vi "Drive Controller.vi"(8 "error in":errorcluster) -> ()   [LabVIEW 2017]
doc: "This VI executes continuously carrying out the current operation and responding to updates or new operation requests. It will often contain the timing or control code that is difficult to place directly in TeleOp. This VI generally opens all sensors and motors and isolates the rest of the robot code from knowing implementation details of how the operations are carried out."
uses:
  <vilib>/Rock Robotics/WPI/Framework/Completion Status.ctl
  Drive Setpoints.ctl
  Drive Operations.ctl
  <vilib>/Rock Robotics/WPI/SafetyOutput/WPI_SafetyOutputConfigMenu.ctl
  <vilib>/Rock Robotics/SystemInterfaces/DIO/FPGA_DIOPWMChannel.ctl
  <vilib>/Rock Robotics/SystemInterfaces/DIO/FPGA_DIOChannel.ctl
  <vilib>/Rock Robotics/WPI/RobotDrive/WPI_RobotDriveOpen2MotorWithTalon.vi
  <vilib>/Rock Robotics/WPI/Counter/WPI_CounterDigitalInputToDigitalSource.vi
  gyroNumControl.vi
  <vilib>/addons/control/pid/pid.llb/PID (DBL).vi
  <vilib>/Rock Robotics/WPI/Joystick/WPI_JoystickArcadeMapping.vi
  <vilib>/addons/control/pid/NI_PID_pid.lvlib
panel:
  in  "PID Gains (DriveDistance)":T1={"proportional gain (Kc)"=1.0, "integral time (Ti, min)"=0.01, "derivative time (Td, min)"=0.0} {"derivative time (Td, min)" format="%.3f"; "integral time (Ti, min)" format="%.3f"; "proportional gain (Kc)" format="%.3f"}
  in  "PID Gains (TurnAngle)":T1={"proportional gain (Kc)"=1.0, "integral time (Ti, min)"=0.01, "derivative time (Td, min)"=0.0} {"derivative time (Td, min)" format="%.3f"; "integral time (Ti, min)" format="%.3f"; "proportional gain (Kc)" format="%.3f"}
  in  "PID gains (GuidedDrive)":T1={"proportional gain (Kc)"=0.1, "integral time (Ti, min)"=0.0, "derivative time (Td, min)"=0.0} {"derivative time (Td, min)" format="%.3f"; "integral time (Ti, min)" format="%.3f"; "proportional gain (Kc)" format="%.3f"}
  in  "Interactive Values":T2
  in  "Buttons":cluster{"Execute Cmd":bool, "Abort Cmd":bool}
  out "Command Timing":cluster{"Start Time (ms)":u32, "Iterations":i32}
  out "Status":T4
  out "Setpoints":T5(graph)
  out "Current\nCmd":string
  # "Tip: The graph shows the motor setpoints. It may also be helpful to observe inputs and sensor values.\nYou may also want to display tuning or debugging controls."
  # "Interactive Command: You may fill in the settings for a command\nand schedule it with the Execute button. You can observe and abort\nany command while fine tuning the code for the controller."
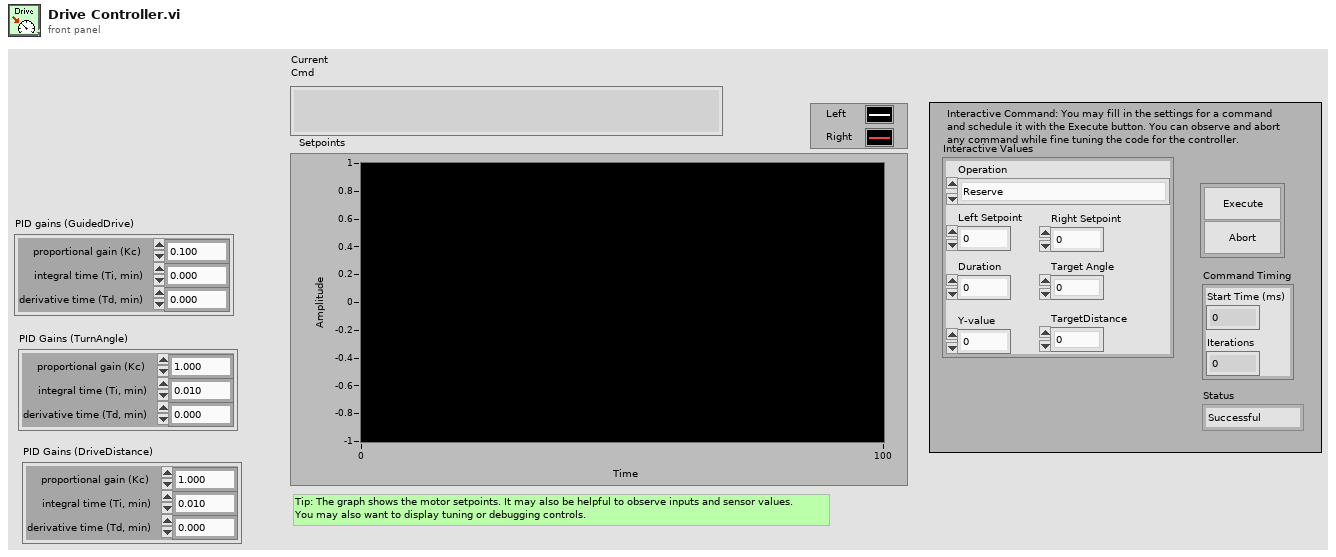
[diagram p1: front panel]
types:
  T1 = cluster{"proportional gain (Kc)":dbl, "integral time (Ti, min)":dbl, "derivative time (Td, min)":dbl}
  T2 = typedef "Drive Setpoints.ctl" = cluster{"Operation":T3, "Left Setpoint":dbl, "Right Setpoint":dbl, "Duration":dbl, "Target Angle":dbl, "Y-value":dbl, "TargetDistance":dbl}
  T3 = typedef "Drive Operations.ctl" = enum16{"Reserve", "Read Current", "Freestyle", "Drive for Distance", "TurnAngle", "Guided Drive"}
  T4 = typedef "Completion Status.ctl" = enum16{"Successful", "Aborted", "Incomplete"}
  T5 = cluster{"Left Setpoint":dbl, "Right Setpoint":dbl}
  T6 = typedef "FPGA_DIOChannel.ctl" = enum8{"DIO 0", "DIO 1", "DIO 2", "DIO 3", "DIO 4", "DIO 5", "DIO 6", "DIO 7", "DIO 8", "DIO 9", "DIO MXP 0", "DIO MXP 1", "DIO MXP 2", "DIO MXP 3", "DIO MXP 4", "DIO MXP 5", "DIO MXP 6", "DIO MXP 7", "DIO MXP 8", "DIO MXP 9", "DIO MXP 10", "DIO MXP 11", "DIO MXP 12", "DIO MXP 13", "DIO MXP 14", "DIO MXP 15", "SPI Port CS1", "SPI Port CS2", "SPI Port CS3", "SPI Port MISO", "SPI Port MOSI", "Invalid"}
  T7 = typedef "FPGA_DIOPWMChannel.ctl" = enum8{"PWM 0", "PWM 1", "PWM 2", "PWM 3", "PWM 4", "PWM 5", "PWM 6", "PWM 7", "PWM 8", "PWM 9", "PWM MXP 0", "PWM MXP 1", "PWM MXP 2", "PWM MXP 3", "PWM MXP 4", "PWM MXP 5", "PWM MXP 6", "PWM MXP 7", "PWM MXP 8", "PWM MXP 9", "Invalid"}
  T8 = typedef "WPI_SafetyOutputConfigMenu.ctl" = enum16{"Enable", "Disable"}
  T9 = typedef "WPI_DigitalInputDevRef.ctl" = cluster{"DevStatus":errorcluster, "DIO Channel":T6}
  T10 = typedef "FPGA_CounterEncoderSourceConvertionLVSourceType.ctl" = cluster{"DevStatus":errorcluster, "AnalogTriggerMode?":bool, "DigitalMode":cluster{"DIO Channel":T11}, "AnalogTriggerMode":cluster{"AnalogTriggerIndex":T12, "OutputType":T13}}
  T11 = typedef "FPGA_DIODigitalSourceChannel.ctl" = enum8{"DIO 0", "DIO 1", "DIO 2", "DIO 3", "DIO 4", "DIO 5", "DIO 6", "DIO 7", "DIO 8", "DIO 9", "DIO MXP 0", "DIO MXP 1", "DIO MXP 2", "DIO MXP 3", "DIO MXP 4", "DIO MXP 5", "DIO MXP 6", "DIO MXP 7", "DIO MXP 8", "DIO MXP 9", "DIO MXP 10", "DIO MXP 11", "DIO MXP 12", "DIO MXP 13", "DIO MXP 14", "DIO MXP 15", "Disabled"}
  T12 = typedef "FPGA_AnalogTriggerIndex.ctl" = enum8{"Trig 0", "Trig 1", "Trig 2", "Trig 3", "Trig 4", "Trig 5", "Trig 6", "Trig 7", "Invalid"}
  T13 = typedef "FPGA_AnalogTriggerOutType.ctl" = enum16{"InWindow", "TriggerState", "Rising", "Falling"}
  T14 = typedef "WPI_RobotDriveDevRef.ctl" = cluster{"DevStatus":errorcluster, "Motors[]":T15[], "Square Inputs":bool, "Max Output":dbl}
  T15 = typedef "WPI_MotorControlDeviceRef.ctl" = cluster{"DeviceStatus":errorcluster, "Type":T16, "PWM":cluster{"PWM Channel":T7, "DeadBand":T17}, "CAN":cluster{"Device Number":u8, "SetOutput VI Ref":variant, "GetOutput VI Ref":variant, "Enable VI Ref":variant, "Disable VI Ref":variant, "Data":variant}, "Invert":bool, "DIO PWM":cluster{"PWM \"Enable\" Channel":T7, "DIOChannel":T6, "PWM Rate":dbl}}
  T16 = typedef "WPI_MotorControlType.ctl" = enum16{"PWM", "CAN", "DIO PWM"}
  T17 = typedef "WPI_PWMDeadband.ctl" = cluster{"Name":string, "maxPositivePwm":i32, "minPositivePwm":i32, "centerPwm":i32, "maxNegativePwm":i32, "minNegativePwm":i32, "angularRange":u16}
  T18 = typedef "WPI_EncoderDevRef.ctl" = cluster{"DevStatus":errorcluster, "EncoderIndex":T19, "CounterIndex":T20, "DistancePerCount":dbl, "Decoding Type":T21}
  T19 = typedef "FPGA_EncoderIdx.ctl" = enum8{"Enc 0", "Enc 1", "Enc 2", "Enc 3", "Enc 4", "Enc 5", "Enc 6", "Enc 7", "Invalid"}
  T20 = typedef "FPGA_CounterCtrSystemIndex.ctl" = enum8{"Ctr 0", "Ctr 1", "Ctr 2", "Ctr 3", "Ctr 4", "Ctr 5", "Ctr 6", "Ctr 7", "Invalid"}
  T21 = typedef "WPI_EncoderType.ctl" = enum16{"1x", "2x", "4x"}
  T22 = typedef "Command Status Info.ctl" = cluster{"Name":string, "Status":T4, "notifier out":T23}
  T23 = typedef "Completion Notifier.ctl" = refnum<notifier>
  T24 = cluster{"SubSystem Data":T2, cluster{"Start Time (ms)":u32, "Iterations":i32}, cluster{"Command Info":T22, "Description":string, "Default Command":T2, "queue out":refnum<queue>, "Subsystem Name":string}}
  T25 = cluster{"SubSystem Data":T2, cluster{"Start Time (ms)":u32, "Iterations":i32}, "Default Command Arguments":cluster{"Command Info":T22, "Description":string, "Default Command":T2, "queue out":refnum<queue>, "Subsystem Name":string}}
  T26 = cluster{"Left Motor Value":dbl, "Right Motor Value":dbl}
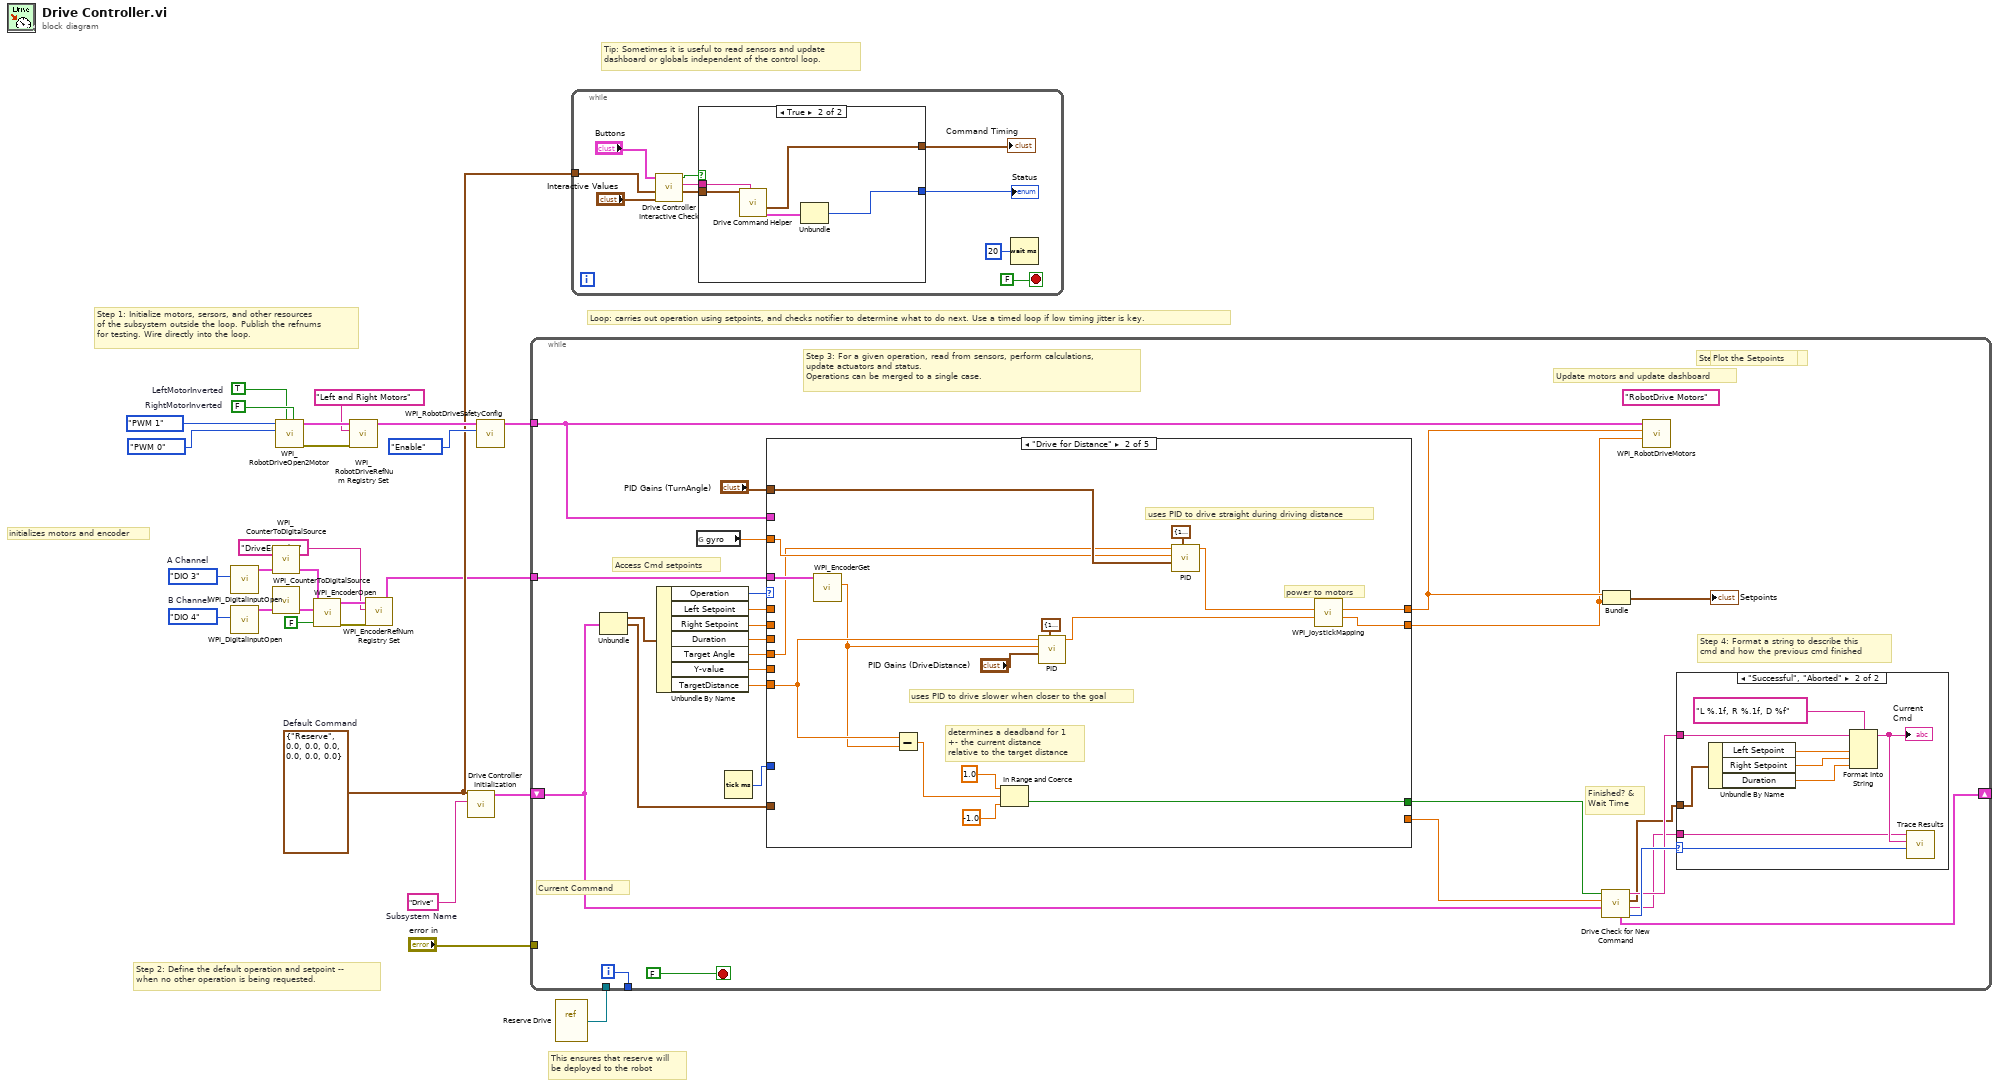
[diagram p0: block diagram]
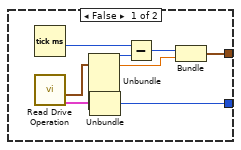
[diagram p2: hidden frame]
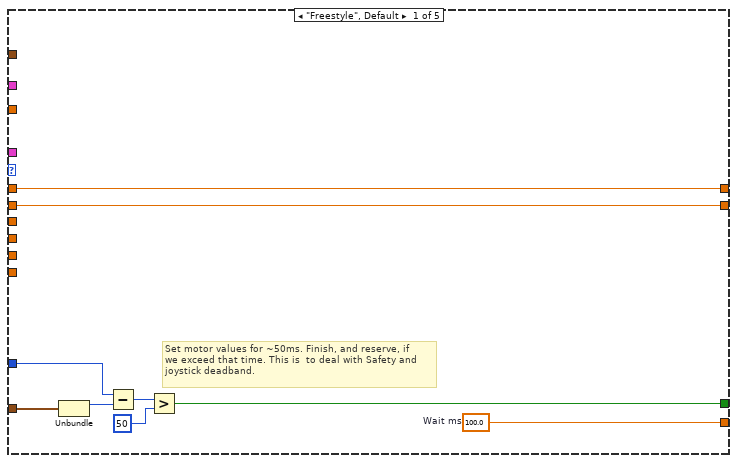
[diagram p4: hidden frame]
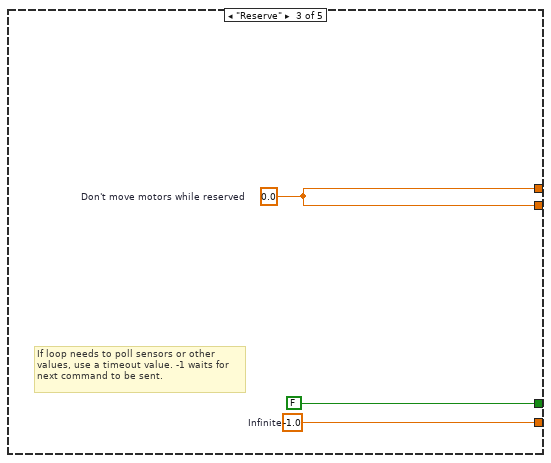
[diagram p5: hidden frame]
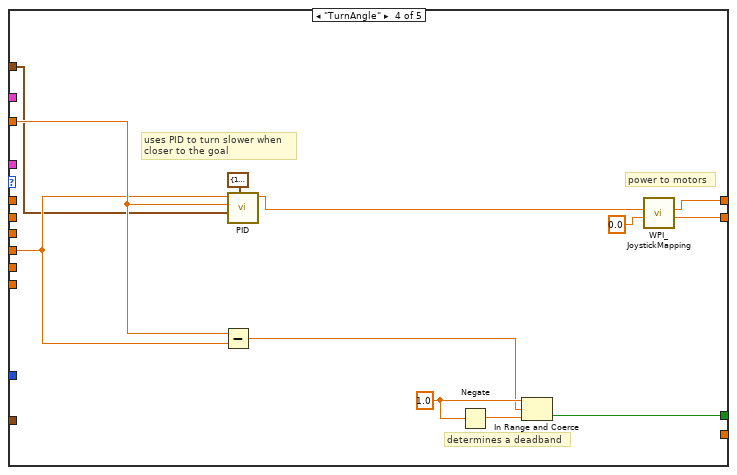
[diagram p6: hidden frame]
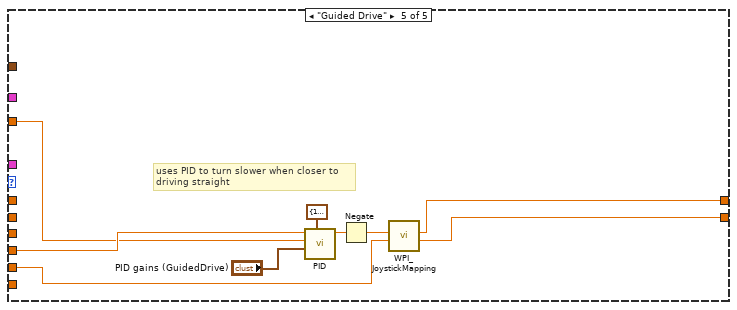
[diagram p7: hidden frame]
diagram:
  w11 = FPGA_DIOChannel."DIO 4"  # B Channel
  w10 = FPGA_DIOChannel."DIO 3"  # A Channel
  w24 = TRUE  # LeftMotorInverted
  w25 = FALSE  # RightMotorInverted
  w12 = T2 {"Operation"=enum."Reserve", "Left Setpoint"=0.0, "Right Setpoint"=0.0, "Duration"=0.0, "Target Angle"=0.0, "Y-value"=0.0, "TargetDistance"=0.0}  # Default Command
  w26 = "Drive"  # Subsystem Name
  # "initializes motors and encoder"
  # "This ensures that reserve will\nbe deployed to the robot"
  # "Tip: Sometimes it is useful to read sensors and update\ndashboard or globals independent of the control loop."
  # "Step 2: Define the default operation and setpoint --\nwhen no other operation is being requested."
  # "Step 1: Initialize motors, sersors, and other resources\nof the subsystem outside the loop. Publish the refnums\nfor testing. Wire directly into the loop."
  # "Loop: carries out operation using setpoints, and checks notifier to determine what to do next. Use a timed loop if low timing jitter is key."
  n1 = call <vilib>:"WPI_DigitalInputOpen.vi"("DIO Channel"=w10) -> ("DigitalInputDevRef"=w7:T9)  [unwired: 1 in, 9 out]
  n2 = call <vilib>:"WPI_DigitalInputOpen.vi"("DIO Channel"=w11) -> ("DigitalInputDevRef"=w8:T9)  [unwired: 1 in, 9 out]
  n3 = call-poly <vilib>:"WPI_CounterToDigitalSource.vi"("DigitalInputDevRef"=w7) -> ("Digital Source"=w6:T10)  [unwired: 6 out]
  n4 = call-poly <vilib>:"WPI_CounterToDigitalSource.vi"("DigitalInputDevRef"=w8) -> ("Digital Source"=w9:T10)  [unwired: 6 out]
  n5 = call-poly <vilib>:"WPI_RobotDriveOpen2Motor.vi"("Right Motor Inverted"=w25, "Left Motor Inverted"=w24, "Right Motor"=FPGA_DIOPWMChannel."PWM 0", "Left Motor"=FPGA_DIOPWMChannel."PWM 1") -> ("error out"=w21:errorcluster, "RobotDriveDevRef"=w23:T14)  [unwired: 1 in, 5 out]
  n6 = call <vilib>:"WPI_EncoderOpen.vi"("Invert Direction (False)"=FALSE, "BSource"=w9, "ASource"=w6) -> ("error out"=w4:errorcluster, "EncoderDevRef"=w3:T18)  [unwired: 5 in, 2 out]
  n7 = call <vilib>:"WPI_RobotDriveRefNum Registry Set.vi"("error in (no error)"=w21, "refnum name"="Left and Right Motors", "RobotDriveDevRef"=w23) -> ("RobotDriveDevRef"=w20:T14)  [unwired: 1 in, 7 out]
  n8 = call <vilib>:"WPI_EncoderRefNum Registry Set.vi"("error in (no error)"=w4, "refnum name"="DriveEncoder", "EncoderDevRef"=w3) -> ("EncoderDevRef"=w2:T18)  [unwired: 7 in, 1 out]
  n9 = call "Drive Controller Initialization.vi"("Subsystem Name"=w26, "Default Command"=w12) -> ("Current Command"=w16:T24)  [unwired: 9 in]
  n10 = call <vilib>:"WPI_RobotDriveSafetyConfig.vi"("mode"=WPI_SafetyOutputConfigMenu."Enable", "RobotDriveDevRef"=w20) -> ("RobotDriveDevRef"=w18:T14)  [unwired: 8 in, 1 out]
  n11 = vi-ref "Reserve Drive.vi"() -> (w15:refnum<vi>)
  n12 = while {
    shift-right: [w41] -> _
    shift-left: w16 -> [w35]
    tunnel: [w52] -> _
    tunnel: w18 -> [w34]
    tunnel: "error in" -> [_]
    tunnel: w15 -> [_]
    tunnel: w2 -> [w29]
    i -> [w52]
    stop <- FALSE stop-if-true
    (unwired) "RobotDrive Motors" ("Name")
    # "Step 5: Upate your I/O"
    # "Step 4: Format a string to describe this\ncmd and how the previous cmd finished"
    # "Current Command"
    # "Update motors and update dashboard"
    # "Plot the Setpoints"
    # "Access Cmd setpoints"
    # "Finished? &\nWait Time"
    # "Step 3: For a given operation, read from sensors, perform calculations,\nupdate actuators and status.\nOperations can be merged to a single case."
    n13 = Unbundle(w35) -> ("SubSystem Data"=w48:T2, w36:cluster{"Start Time (ms)":u32, "Iterations":i32})  [unwired: 1 out]
    n14 = Unbundle By Name(w48) -> ("Operation"=w47:T3, "Left Setpoint"=w46:dbl, "Right Setpoint"=w45:dbl, "Duration"=w44:dbl, "Target Angle"=w30:dbl, "Y-value"=w31:dbl, "TargetDistance"=w28:dbl)
    n15 = global read "gyroNumControl.vi" "gyro"() -> (w32:dbl)
    n16 = Tick Count (ms)() -> (millisecond timer value=w43:u32)
    n17 = case shown="\"Drive for Distance\"" w47 {
      tunnel: [w71 _ w91 _ _] -> w40
      tunnel: [w64 w84 FALSE ("ignore previous (F)") w103 _] -> w33
      tunnel: w36 -> [w63 _ _ _ _]
      tunnel: [w70 w76 w89 w102 w107] -> w50
      tunnel: [w69 w75 w89 w101 w105] -> w49
      tunnel: w46 -> [w70 _ _ _ _]
      tunnel: w45 -> [w69 _ _ _ _]
      tunnel: w44 -> [_ _ _ _ _]
      tunnel: w43 -> [w65 _ _ _ _]
      tunnel: w34 -> [_ _ _ _ _]
      tunnel: w32 -> [_ w73 _ w98 w111]
      tunnel: w31 -> [_ _ _ _ w106]
      tunnel: w30 -> [_ w72 _ w97 w112]
      tunnel: w29 -> [_ w88 _ _ _]
      tunnel: w28 -> [_ w83 _ _ _]
      tunnel: "PID Gains (TurnAngle)" -> [_ w77 _ w92 _]
      frame "Freestyle", Default {
        w71 = 100.0  # Wait ms
        # "Set motor values for ~50ms. Finish, and reserve, if\nwe exceed that time. This is  to deal with Safety and\njoystick deadband."
        n18 = Unbundle(w63) -> ("Start Time (ms)"=w66:u32)  [unwired: 1 out]
        n19 = Subtract(x=w65, y=w66) -> (x-y=w67:u32)
        n20 = Greater?(x=w67, y=u8 50 ("Left Motor")) -> (0:w64:bool)
      }
      frame "Drive for Distance" {
        # "uses PID to drive straight during driving distance"
        # "power to motors"
        # "uses PID to drive slower when closer to the goal"
        # "determines a deadband for 1\n+- the current distance \nrelative to the target distance"
        n21 = call <vilib>:"WPI_EncoderGet.vi"("EncoderDevRef"=w88) -> ("Distance"=w82:dbl)  [unwired: 5 in, 5 out]
        n22 = Subtract(x=w83, y=w82) -> (x-y=w87:dbl)
        n23 = In Range and Coerce(upper limit=1.0, x=w87, lower limit=-1.0) -> (In Range?=w84:bool)  [unwired: 1 out]
        n24 = call-poly <vilib>:"PID.vi"("output range"=cluster{"output high":dbl, "output low":dbl} {"output high"=1.0, "output low"=-1.0}, "PID gains"="PID Gains (DriveDistance)", "process variable"=w82, "setpoint"=w83) -> ("output"=w74:dbl)  [unwired: 6 in, 1 out]
        n25 = call-poly <vilib>:"PID.vi"("output range"=cluster{"output high":dbl, "output low":dbl} {"output high"=1.0, "output low"=-1.0}, "PID gains"=w77, "process variable"=w73, "setpoint"=w72) -> ("output"=w78:dbl)  [unwired: 6 in, 1 out]
        n26 = call-poly <vilib>:"WPI_JoystickMapping.vi"("Y axis value"=w74, "X axis value"=w78) -> ("Right Motor Value"=w75:dbl, "Left Motor Value"=w76:dbl)  [unwired: 8 in]
      }
      frame "Reserve" {
        w89 = 0.0  # Don't move motors while reserved
        w91 = -1.0  # Infinite
        # "If loop needs to poll sensors or other\nvalues, use a timeout value. -1 waits for\nnext command to be sent."
      }
      frame "TurnAngle" {
        w99 = 1.0 ("x")
        # "power to motors"
        # "uses PID to turn slower when\ncloser to the goal"
        # "determines a deadband"
        n27 = Subtract(x=w98, y=w97) -> (x-y=w96:dbl)
        n28 = call-poly <vilib>:"PID.vi"("output range"=cluster{"output high":dbl, "output low":dbl} {"output high"=1.0, "output low"=-1.0}, "PID gains"=w92, "process variable"=w98, "setpoint"=w97) -> ("output"=w94:dbl)  [unwired: 6 in, 1 out]
        n29 = Negate(x=w99) -> (-x=w100:dbl)
        n30 = In Range and Coerce(upper limit=w99, x=w96, lower limit=w100) -> (In Range?=w103:bool)  [unwired: 1 out]
        n31 = call-poly <vilib>:"WPI_JoystickMapping.vi"("Y axis value"=0.0, "X axis value"=w94) -> ("Right Motor Value"=w101:dbl, "Left Motor Value"=w102:dbl)  [unwired: 8 in]
      }
      frame "Guided Drive" {
        # "uses PID to turn slower when closer to\ndriving straight"
        n32 = call-poly <vilib>:"PID.vi"("output range"=cluster{"output high":dbl, "output low":dbl} {"output high"=1.0, "output low"=-1.0}, "PID gains"="PID gains (GuidedDrive)", "process variable"=w111, "setpoint"=w112) -> ("output"=w108:dbl)  [unwired: 6 in, 1 out]
        n33 = Negate(x=w108) -> (-x=w104:dbl)
        n34 = call-poly <vilib>:"WPI_JoystickMapping.vi"("Y axis value"=w106, "X axis value"=w104) -> ("Right Motor Value"=w105:dbl, "Left Motor Value"=w107:dbl)  [unwired: 8 in]
      }
    }
    n35 = call "Drive Check for New Command.vi"("input cluster"=w35, "Wait time (ms)"=w40, "Finished?"=w33) -> ("Completion"=w42:T4, "Subsystem Name"=w37:string, "Current Command"=w38:T2, "Initial Trace String"=w39:string, "Next Command"=w41:T25)  [unwired: 4 in]
    n36 = Bundle("Left Motor Value"=w50, "Right Motor Value"=w49) -> (→"Setpoints":T26)  [unwired: 1 in]
    n37 = call <vilib>:"WPI_RobotDriveMotors.vi"("RightSpeed"=w49, "LeftSpeed"=w50, "RobotDriveDevRef"=w34) -> ()  [unwired: 1 in, 8 out]
    n38 = case shown="\"Successful\", \"Aborted\"" w42 {
      selector: w42 -> [_ w62]
      tunnel: w39 -> [_ w57]
      tunnel: w38 -> [_ w58]
      tunnel: w37 -> [_ w54]
      frame "Incomplete", Default {
        # "Continuing current command"
      }
      frame "Successful", "Aborted" {
        # "Report and setup for next command"
        n39 = Unbundle By Name(w58) -> ("Left Setpoint"=w60:dbl, "Right Setpoint"=w61:dbl, "Duration"=w55:dbl)
        n40 = Format Into String(format string="L %.1f, R %.1f, D %f", initial string=w57, w60, w61, w55) -> (resulting string=w56:string)  [unwired: 1 in, 1 out]
        "Current\nCmd" <- w56
        n41 = call <vilib>:"Trace Results.vi"("Status of previous command"=w62, "Description"=w56, "Subsystem"=w54) -> ()  [unwired: 9 in]
      }
    }
  }
  n42 = while {
    tunnel: w12 -> [w114]
    stop <- FALSE stop-if-true
    n43 = call "Drive Controller Interactive Check.vi"("Interactive Command In"="Interactive Values", "Default Command"=w114, "Buttons"="Buttons") -> ("Interactive Command Out"=w116:T2, "Trace String"=w117:string, "Schedule"=w118:bool)  [unwired: 6 in]
    n44 = case shown="True" w118 {
      tunnel: [w127 w135] -> w119
      tunnel: [w126 w131] -> w120
      tunnel: w117 -> [_ w133]
      tunnel: w116 -> [_ w132]
      frame False {
        n45 = Tick Count (ms)() -> (millisecond timer value=w130:u32)
        n46 = call "Read Drive Operation.vi"() -> ("Command Info"=w124:T22, "SubSystem Data"=w123:T2)  [unwired: 9 in, 1 out]
        n47 = Unbundle(w123) -> ("Operation"=w128:T3, "Left Setpoint"=w125:dbl)  [unwired: 5 out]
        n48 = Unbundle(w124) -> ("Status"=w127:T4)  [unwired: 2 out]
        n49 = Subtract(x=w130, y=w128) -> (x-y=w129:u32)
        n50 = Bundle(w129, "Left Setpoint"=w125) -> (w126:cluster{u32, "Left Setpoint":dbl})  [unwired: 1 in]
      }
      frame True {
        n51 = call "Drive Command Helper.vi"("Description"=w133, "SubSystem Data"=w132) -> ("Command Info Out"=w134:T22, "Command Timing"=w131:cluster{"Start Time (ms)":u32, "Iterations":i32})  [unwired: 7 in, 1 out]
        n52 = Unbundle(w134) -> ("Status"=w135:T4)  [unwired: 2 out]
      }
    }
    "Status" <- w119
    "Command Timing" <- w120
    n53 = Wait (ms)(milliseconds to wait=u32 20) -> ()  [unwired: 1 out]
  }
